vi "getVariableHeaderLength.vi"(11 "CONNACK in":refnum<class "CONNACK.lvclass">) -> (1 "size definitive":bool, 2 "VariableHeader size":u32, 3 "CONNACK out":refnum<class "CONNACK.lvclass">)   [LabVIEW 2013, in "MQTT_Control_Packets.lvlib" / "CONNACK.lvclass"]
uses:
  CONNACK.lvclass
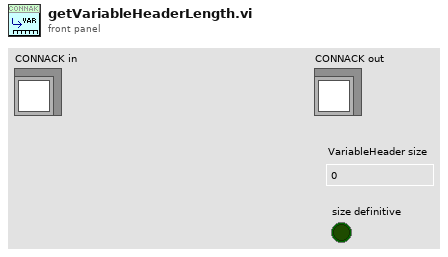
[diagram p1: front panel]
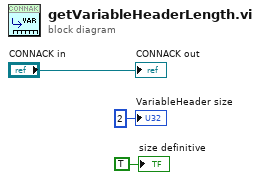
[diagram p0: block diagram]
diagram:
  "CONNACK out" <- "CONNACK in"
  "VariableHeader size" <- u32 2 ("VariableHeader size")
  "size definitive" <- TRUE ("size definitive")
